vi "Mode Value.vi"(1 "Mode In":T1(ring)=enum."Train", 2 "Read/Write this vi":bool) -> (0 "Mode Out":T1(ring))   [LabVIEW 2024]
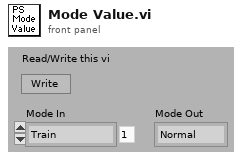
[diagram p1: front panel]
types:
  T1 = enum16{"Normal", "Train", "Lambda", "Train & Lambda"}
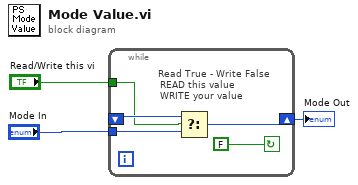
[diagram p0: block diagram]
diagram:
  n1 = while {
    tunnel: "Read/Write this vi" -> [w4]
    shift-right: [w6] -> w1
    shift-left: _ -> [w5]
    tunnel: "Mode In" -> [w7]
    stop <- FALSE continue-if-true
    # "READ this value\nWRITE your value"
    # "Read True - Write False"
    n2 = Select(t=w5, s=w4, f=w7) -> (s? t:f=w6:T1)
  }
  "Mode Out" <- w1
